vi "GetDeviceTypeConfig.vi"(8 "error in (no error)":errorcluster) -> (0 "error out":errorcluster, 1 "found":bool, 3 "key values":T1[](array[typedef]))   [LabVIEW 2017, in "GlobalConfiguration.lvlib"]
doc: "Returns various global properties designed to control certain behaviors in processes. These properties affect behaviors that you do not need users to customize on a per-device basis. For example, one NI-developed property defines how often the File Manager process evaluates its free disk space to ensure a minimum amount remains free."
uses:
  <vilib>/addons/InsightCM/Utilities/GlobalConfiguration/GlobalConfiguration.lvlib
  <vilib>/addons/InsightCM/MessageBus/Base/controls/SectionKeyValues.ctl
  <vilib>/addons/InsightCM/MessageBus/Base/controls/KeyValuePair.ctl
  <vilib>/addons/PointValueMap/subVIs/Point_Read_variant.vi
  <vilib>/addons/PointValueMap/subVIs/Point_Write_variant.vi
  <vilib>/addons/PointValueMap/PointValueMap.lvlib
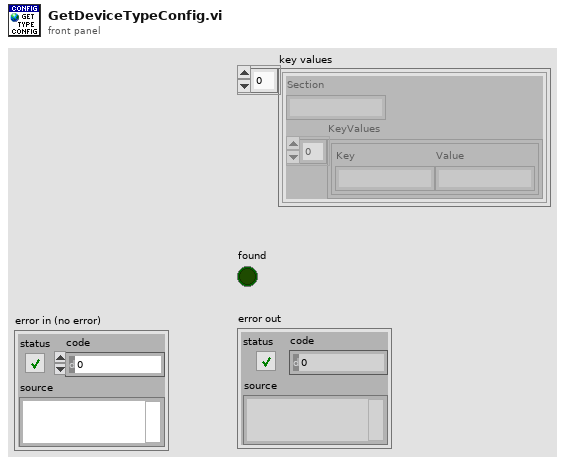
[diagram p1: front panel]
types:
  T1 = typedef "SectionKeyValues.ctl" = cluster{"Section":string, "KeyValues":T2[]}
  T2 = typedef "KeyValuePair.ctl" = cluster{"Key":string, "Value":string}
  T3 = typedef "PointValueMap.lvlib/PointMap.ctl" = refnum<data-value>
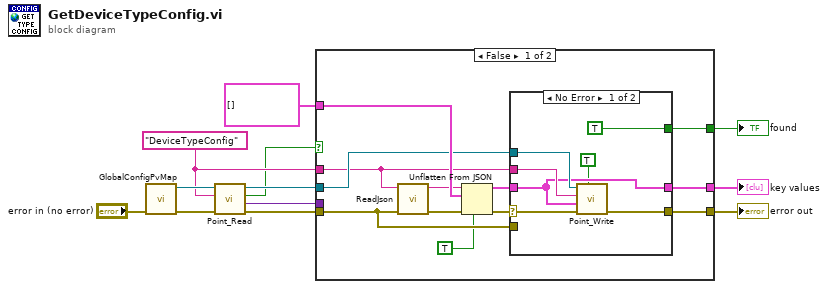
[diagram p0: block diagram]
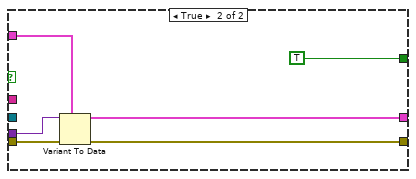
[diagram p3: hidden frame]
diagram:
  w7 = "DeviceTypeConfig" ("Name")
  n1 = call <vilib>:"GlobalConfigPvMap.vi"("error in (no error)"="error in (no error)") -> ("error out"=w9:errorcluster, "global configuration map"=w10:T3)  [unwired: 9 in]
  n2 = call-poly <vilib>:"Point_Read.vi"("Error In"=w9, "Tag"=w7, "Map"=w10) -> ("Error Out"=w4:errorcluster, "Value"=w5:variant, "Found?"=w3:bool, "Map Out"=w6:T3)  [unwired: 3 in, 2 out]
  n3 = case shown="False" w3 {
    tunnel: [w15 w38] -> w12
    tunnel: [w16 w37] -> w1
    tunnel: [w20 TRUE] -> w8
    tunnel: w7 -> [w18 _]
    tunnel: T1[] [] ("KeyValues") -> [w23 w35]
    tunnel: w6 -> [w19 _]
    tunnel: w5 -> [_ w34]
    tunnel: w4 -> [w14 w33]
    frame False {
      n4 = call <vilib>:"ReadJson.vi"("error in (no error)"=w14, "json object"=w18) -> ("error out"=w24:errorcluster, "json string"=w22:string)  [unwired: 8 in]
      n5 = Unflatten From JSON(JSON string=w22, type and defaults=w23, default null elements? (F)=TRUE, error in (no error)=w24) -> (value=w17:T1[], error out=w21:errorcluster)  [unwired: 3 in]
      n6 = case shown="No Error" w21 {
        selector: w21 -> [w31 _]
        tunnel: [TRUE _] -> w20
        tunnel: w19 -> [w29 _]
        tunnel: w18 -> [w28 _]
        tunnel: w17 -> [w27 _]
        tunnel: [w27 _] -> w16
        tunnel: [w26 w32] -> w15
        tunnel: w14 -> [_ w32]
        frame No Error {
          n7 = call-poly <vilib>:"Point_Write.vi"("Auto Create?"=TRUE, "Error In"=w31, "Value"=w27, "Tag"=w28, "Map"=w29) -> ("Error Out"=w26:errorcluster)  [unwired: 5 in, 1 out]
        }
        frame Error {
        }
      }
    }
    frame True {
      n8 = Variant To Data(error in=w33, type=w35, Variant=w34) -> (data=w37:T1[], error out=w38:errorcluster)
    }
  }
  "error out" <- w12
  "found" <- w8
  "key values" <- w1
